vi "build.vi"(8 "error in (no error)":errorcluster, 10 "build_spec":T1, 11 "lv-build-default in":refnum<class "lv-builder-default.lvclass">) -> (0 "error out":errorcluster, 2 "[] generated_files":path[](array[path]), 3 "lv-build-default out":refnum<class "lv-builder-default.lvclass">)   [LabVIEW 2015, in "lv-builder-default.lvclass"]
uses:
  lv-builder-default.lvclass
  lv-build/public/_controls/build_specification.ctl
  lv-build/public/_controls/build_type.ctl
  community/_controls/configuration.ctl
  <vilib>/AppBuilder/AB_API_Simple/Set Build Specification Version (path).vi
  lv-builder-default.lvlib
  <vilib>/AppBuilder/AB_API_Simple/NI_App_Builder_API.lvlib
  lv-build/lv-build.lvlib
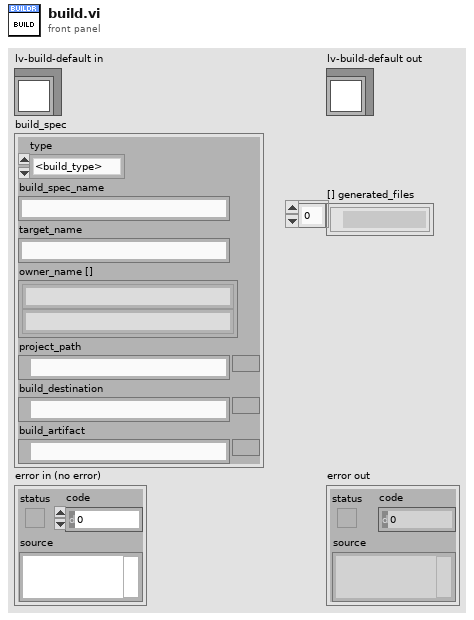
[diagram p1: front panel]
types:
  T1 = typedef "lv-build.lvlib/build_specification.ctl" = cluster{"type":T2, "build_spec_name":string, "target_name":string, "owner_name []":string[], "project_path":path, "build_destination":path, "build_artifact":path}
  T2 = typedef "lv-build.lvlib/build_type.ctl" = enum16{"<build_type>", "application_pc", "application_rt", "installer", "llb", "lvlibp", "zip", "fpga", "<null>"}
  T3 = typedef "lv-builder-default.lvlib/configuration.ctl" = cluster{"project_file":string, "lvlibp_directory":string, "zip_directory":string, "lvlib_directory":string, "update_version_vi":string, "installer_post_file":string, "distribution_folder":string, "dependencies_folder":string, "version":string, "bin_folder":string, "lvlib_post_action":u16, "installer_post_action":u16, "application_post_action":u16, "zip_post_action":u16}
  T4 = typedef "NI_App_Builder_API.lvlib/Build Specification Version.ctl" = cluster{"Major":u16, "Minor":u16, "Fix":u16, "Build":u16}
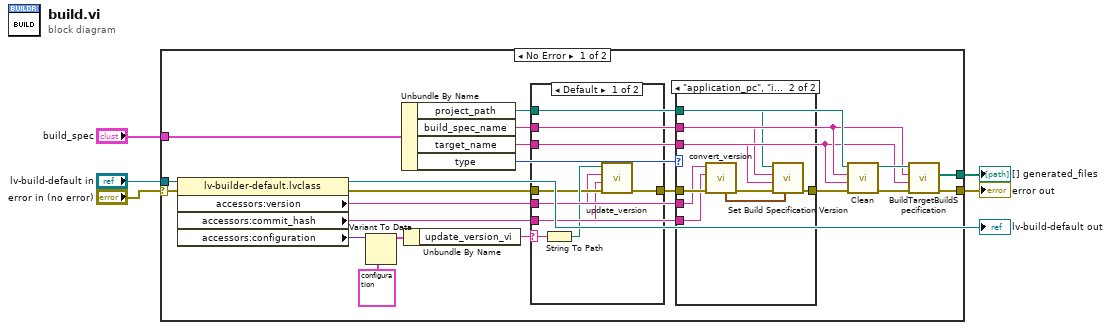
[diagram p0: block diagram]
diagram:
  n1 = case shown="No Error" "error in (no error)" {
    selector: "error in (no error)" -> [w19 w42]
    tunnel: [w21 w42] -> w3
    tunnel: "lv-build-default in" -> [w18 _]
    tunnel: "build_spec" -> [w23 _]
    tunnel: [w20 _] -> w2
    frame No Error {
      n2 = property class="lv-builder-default.lvclass"(reference=w18, error in=w19) -> (error out=w14:errorcluster, "accessors:version"=w11:string, "accessors:commit_hash"=w12:string, "accessors:configuration"=w17:variant)  [unwired: 1 out]
      n3 = Variant To Data(type=T3 {"project_file"="", "lvlibp_directory"="", "zip_directory"="", "lvlib_directory"="", "update_version_vi"="", "installer_post_file"="", "distribution_folder"="", "dependencies_folder"="", "version"="", "bin_folder"="", "lvlib_post_action"=0, "installer_post_action"=0, "application_post_action"=0, "zip_post_action"=0} ("configuration"), Variant=w17) -> (data=w15:T3)  [unwired: 1 in, 1 out]
      n4 = Unbundle By Name(w23) -> ("project_path"=w10:path, "build_spec_name"=w9:string, "target_name"=w6:string, "type"=w7:T2)
      n5 = Unbundle By Name(w15) -> ("update_version_vi"=w13:string)
      n6 = case shown="Default" w13 {
        selector: w13 -> [w40 _]
        tunnel: [w35 w41] -> w24
        tunnel: w10 -> [_ _]
        tunnel: w9 -> [_ _]
        tunnel: w6 -> [_ _]
        tunnel: w14 -> [w38 w41]
        tunnel: w11 -> [w37 _]
        tunnel: w12 -> [w36 _]
        frame Default {
          n7 = String To Path(string=w40) -> (path=w39:path)
          n8 = call "update_version.vi"("error in (no error)"=w38, "commit_hash"=w36, "version"=w37, "version_vi"=w39) -> ("error out"=w35:errorcluster)  [unwired: 7 in]
        }
        frame "" {
        }
      }
      n9 = case shown="\"application_pc\", \"installer\"" w7 {
        tunnel: w24 -> [w25 w34]
        tunnel: w12 -> [_ w31]
        tunnel: w11 -> [_ w30]
        tunnel: w10 -> [_ w29]
        tunnel: w9 -> [_ w28]
        tunnel: [w25 w27] -> w8
        tunnel: w6 -> [_ w26]
        frame Default {
        }
        frame "application_pc", "installer" {
          n10 = call "convert_version.vi"("error in (no error)"=w34, "version_delimiter"=w31, "version"=w30) -> ("error out"=w33:errorcluster, "build_specification_version"=w32:T4)  [unwired: 7 in]
          n11 = call-poly <vilib>:"Set Build Specification Version.vi"("Build Specification Version"=w32, "error in (no error)"=w33, "Name of target (My Computer)"=w26, "Name of build specification"=w28, "Path to project"=w29) -> ("error out"=w27:errorcluster)  [unwired: 6 in]
        }
      }
      n12 = call <vilib>:"Clean.vi"("error in (no error)"=w8, "Name of target (My Computer)"=w6, "Name of build specification (if empty: clean all)"=w9, "Path to project"=w10) -> ("error out"=w22:errorcluster)  [unwired: 7 in]
      n13 = call <vilib>:"BuildTargetBuildSpecification.vi"("error in (no error)"=w22, "Name of target (My Computer)"=w6, "Name of build specification (if empty: build all)"=w9, "Path to project"=w10) -> ("error out"=w21:errorcluster, "Generated files"=w20:path[])  [unwired: 6 in]
    }
    frame Error {
    }
  }
  "error out" <- w3
  "[] generated_files" <- w2
  "lv-build-default out" <- "lv-build-default in"
